vi "Load Settings from XML.vi"() -> (0 "error out":errorcluster, 3 "Settings out":T1={"Calibration Array"=[], "Hardware Config Cluster"=[], "Trigger Settings"={"Trigger Type"=enum."No Trigger", "Digital Start"={"Source"="", "Digital Start Trigger Edge"=0}, "Digital Pause"={"Source"="APFI0", "Digital Pause Trigger Pause When"=10192}, "Digital Reference"={"Source"="", "Digital Start Trigger Edge"=10280, "Digital Reference Pretrigger Samples"=0}, "Analog Start"={"Source"="", "Analog Slope"=10093, "Analog Start Trigger Hysteresis"=0.0, "Analog Start Trigger Level"=0.0}, "Analog Pause"={"Source"="", "Analog Start Trigger Level"=0.0, "Analog Pause Trigger Pause When"=10093}, "Analog Reference"={"Source"="", "Slope"=10280, "Pretrigger Samples"=0, "Level"=0.0}, "Time Start"={"Select Time\nManually"=FALSE, "When"=timestamp(0 s since 1904-01-01)}}, "Log File Base Path"=path "", "DAQmx Timing Settings"={"rate"=1000.0, "source"="OnboardClock", "sample mode"=10178, "samples per channel"=1000}} {"DAQmx Timing Settings"."sample mode" items=["Finite Samples"=10178, "Continuous Samples"=10123, "Hardware Timed Single Point"=12522]; "DAQmx Timing Settings"."rate" format="%0.2f"; "Trigger Settings"."Time Start"."When" format="%<%x %.3X>T"; "Trigger Settings"."Analog Reference"."Level" format="%0.2f"; "Trigger Settings"."Analog Reference"."Slope" items=["Rising"=10280, "Falling"=10171]; "Trigger Settings"."Analog Pause"."Analog Pause Trigger Pause When" items=["Above Level"=10093, "Below Level"=10107]; "Trigger Settings"."Analog Pause"."Analog Start Trigger Level" format="%0.2f"; "Trigger Settings"."Analog Start"."Analog Start Trigger Level" format="%0.2f"; "Trigger Settings"."Analog Start"."Analog Start Trigger Hysteresis" format="%.2f"; "Trigger Settings"."Analog Start"."Analog Slope" items=["Rising"=10280, "Falling"=10171]; "Trigger Settings"."Digital Reference"."Digital Start Trigger Edge" items=["Rising"=10280, "Falling"=10171]; "Trigger Settings"."Digital Pause"."Digital Pause Trigger Pause When" items=["High"=10192, "Low"=10214]; "Trigger Settings"."Digital Start"."Digital Start Trigger Edge" items=["Rising"=10280, "Falling"=10171]; "Hardware Config Cluster"."Unit" items=["Volts", "From Custom Scale"]})   [LabVIEW 2020, in "Settings Editor.lvlib"]
doc: "Attempts to load previous user specified settings from an XML file.\n\nThis VI will not generate an error. If a suitable XML file can't be loaded and parsed then it will simply return the default settings.\n_____\nBased on DQMH Project Template 6.0.0.91."
uses:
  Settings Editor.lvlib
  Settings--cluster.ctl
  DAQmx Config--cluster.ctl
  DAQmx Trigger Settings--cluster.ctl
  DAQmx Timing--cluster.ctl
  <vilib>/Utility/xml.llb/Read From XML File(string).vi
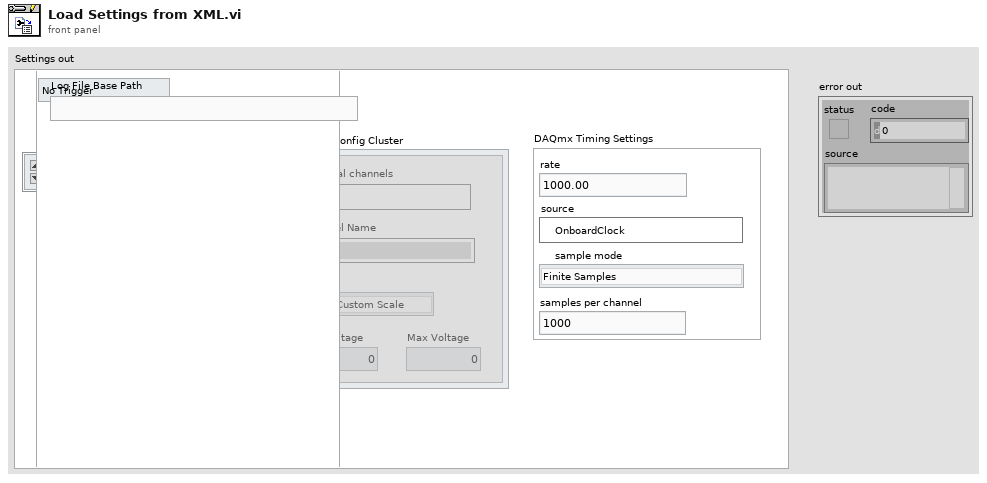
[diagram p1: front panel]
types:
  T1 = typedef "Settings Editor.lvlib/Settings--cluster.ctl" = cluster{"Calibration Array":cluster{"Slope":dbl, "Offset":dbl}[], "Hardware Config Cluster":T2, "Trigger Settings":T3, "Log File Base Path":path, "DAQmx Timing Settings":T4}
  T2 = typedef "Settings Editor.lvlib/DAQmx Config--cluster.ctl" = cluster{"Physical channels":tag, "Channel Name":string, "Unit":i32, "Min Voltage":dbl, "Max Voltage":dbl}[]
  T3 = typedef "Settings Editor.lvlib/DAQmx Trigger Settings--cluster.ctl" = cluster{"Trigger Type":enum32{"No Trigger", "Digital Start", "Digital Pause", "Digital Reference", "Analog Start", "Analog Pause", "Analog Reference", "Time Start"}, "Digital Start":cluster{"Source":tag, "Digital Start Trigger Edge":i32}, "Digital Pause":cluster{"Source":tag, "Digital Pause Trigger Pause When":i32}, "Digital Reference":cluster{"Source":tag, "Digital Start Trigger Edge":i32, "Digital Reference Pretrigger Samples":u32}, "Analog Start":cluster{"Source":string, "Analog Slope":i32, "Analog Start Trigger Hysteresis":dbl, "Analog Start Trigger Level":dbl}, "Analog Pause":cluster{"Source":string, "Analog Start Trigger Level":dbl, "Analog Pause Trigger Pause When":i32}, "Analog Reference":cluster{"Source":string, "Slope":i32, "Pretrigger Samples":u32, "Level":dbl}, "Time Start":cluster{"Select Time\nManually":bool, "When":timestamp}}
  T4 = typedef "Settings Editor.lvlib/DAQmx Timing--cluster.ctl" = cluster{"rate":dbl, "source":tag, "sample mode":i32, "samples per channel":i32}
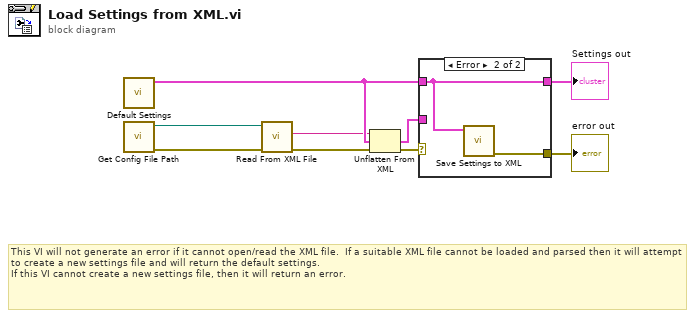
[diagram p0: block diagram]
diagram:
  # "This VI will not generate an error if it cannot open/read the XML file.  If a suitable XML file cannot be loaded and parsed then it will attempt to create a new settings file and will return the default settings.\nIf this VI cannot create a new settings file, then it will return an error."
  n1 = call "Default Settings.vi"() -> ("Default Settings"=w7:T1)  [unwired: 11 in]
  n2 = call "Get Config File Path.vi"() -> ("error out"=w3:errorcluster, "XML File Path"=w4:path)  [unwired: 10 in]
  n3 = call-poly <vilib>:"Read From XML File.vi"("error in (no error)"=w3, "XML File Path"=w4) -> ("error out"=w5:errorcluster, "XML Elements"=w6:string)  [unwired: 7 in, 1 out]
  n4 = Unflatten From XML(xml string=w6, type=w7, error in (no error)=w5) -> (value=w1:T1, error out=w2:errorcluster)
  n5 = case shown="Error" w2 {
    tunnel: [w10 w12] -> w8
    tunnel: w7 -> [_ w12]
    tunnel: w1 -> [w10 _]
    tunnel: [_ w11] -> w9
    frame No Error {
    }
    frame Error {
      n6 = call "Save Settings to XML.vi"("Settings"=w12) -> ("error out"=w11:errorcluster)  [unwired: 10 in]
    }
  }
  "error out" <- w9
  "Settings out" <- w8
